vi "DefaultFromIni.vi"(8 "error in (no error)":errorcluster, 11 "FFT in":refnum<class "FFT.lvclass">) -> (0 "error out":errorcluster, 3 "FFT out":refnum<class "FFT.lvclass">)   [LabVIEW 2018, in "AnalysisPlugins.lvlib" / "FFT.lvclass"]
uses:
  FFT.lvclass
  FitterBaseClass/FitterBase.lvclass
  <vilib>/Utility/config.llb/NI_LVConfig.lvlib
  Typedefs/FftView.ctl
  <vilib>/Analysis/4window.llb/windowTd.ctl
  <vilib>/Analysis/NI_AALPro.lvlib
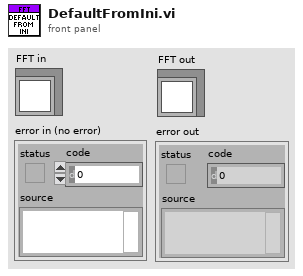
[diagram p1: front panel]
types:
  T1 = typedef "NI_AALPro.lvlib/windowTd.ctl" = u32
  T2 = typedef "AnalysisPlugins.lvlib/FFT.lvclass/FftView.ctl" = cluster{"dB On (F)":bool, "unwrap phase (F)":bool, "convert to degree (F)":bool}
  T3 = typedef "NI_LVConfig.lvlib/Config Data RefNum.ctl" = refnum<k1>
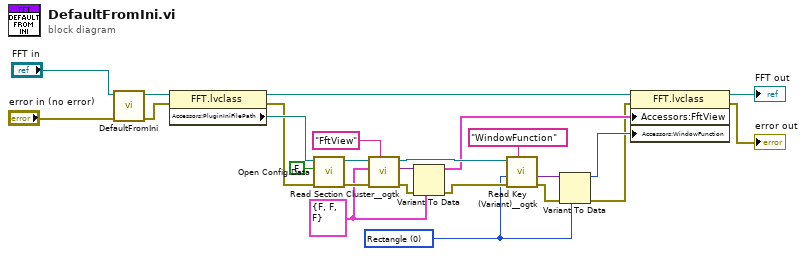
[diagram p0: block diagram]
diagram:
  w4 = T1 0 items=["Rectangle"=0, "Hanning"=1, "Hamming"=2, "Blackman-Harris"=3, "Exact Blackman"=4, "Blackman"=5, "Flat Top"=6, "4 Term B-Harris "=7, "7 Term B-Harris"=8, "Low Sidelobe"=9, "Blackman Nuttall"=11, "Triangle"=30, "Bartlett-Hanning"=31, "Bohman"=32, "Parzen"=33, "Welch"=34, "Kaiser"=60, "Dolph-Chebyshev"=61, "Gaussian"=62] ("WindowFunction")
  w11 = T2 {"dB On (F)"=FALSE, "unwrap phase (F)"=FALSE, "convert to degree (F)"=FALSE} ("FftView")
  n1 = call-parent "DefaultFromIni.vi"("error in (no error)"="error in (no error)", "FitterBase in"="FFT in") -> ("error out"=w21:errorcluster, "FitterBase out"=w25:refnum<class "FFT.lvclass">)  [unwired: 8 in]
  n2 = property class="FFT.lvclass"(reference=w25, error in=w21) -> (reference out=w22:refnum<class "FFT.lvclass">, error out=w18:errorcluster, "Accessors:PluginIniFilePath"=w20:path)
  n3 = call <vilib>:"Open Config Data.vi"("error in (no error)"=w18, "create file if necessary (T)"=FALSE, "configuration file path"=w20) -> ("error out"=w16:errorcluster, "refnum"=w15:T3)  [unwired: 6 in, 1 out]
  n4 = call <userlib>:"Read Section Cluster__ogtk.vi"("section (optional)"="FftView", "error in (no error)"=w16, "Section Formatted Cluster Type"=w11, "refnum"=w15) -> ("error out"=w13:errorcluster, "Section Formatted Cluster"=w12:variant, "dup refnum"=w9:T3)  [unwired: 3 in, 2 out]
  n5 = Variant To Data(error in=w13, type=w11, Variant=w12) -> (data=w8:T2, error out=w10:errorcluster)
  n6 = call <userlib>:"Read Key (Variant)__ogtk.vi"("section"="WindowFunction", "error in (no error)"=w10, "type"=w4, "refnum"=w9) -> ("error out"=w7:errorcluster, "key-value"=w6:variant)  [unwired: 4 in, 2 out]
  n7 = Variant To Data(error in=w7, type=w4, Variant=w6) -> (data=w3:T1, error out=w2:errorcluster)
  n8 = property class="FFT.lvclass"(reference=w22, error in=w2, "Accessors:FftView"=w8, "Accessors:WindowFunction"=w3) -> (reference out=→"FFT out":refnum<class "FFT.lvclass">, error out=→"error out":errorcluster)
